vi "LVClass_HasoData Reset To RAW data.vi"(0 "HasoData in":refnum<class "HasoData.lvclass">, 11 "error in (no error)":errorcluster) -> (4 "HasoData out":refnum<class "HasoData.lvclass">, 15 "error out":errorcluster)   [LabVIEW 2020, in "HasoData.lvclass"]
doc: "Reset slopes to their raw state and clear process history.\n\n--------------------------------------------------------------------------------\n\n<B>HasoDataIn </B> : HasoData object.\n<B>HasoDataOut </B> : HasoData object.\n<B>ErrorIn </B> : Error\n<B>ErrorOut </B> : Error\n\n--------------------------------------------------------------------------------"
uses:
  HasoData.lvclass
  HasoData.lvclass/HasoData.ctl
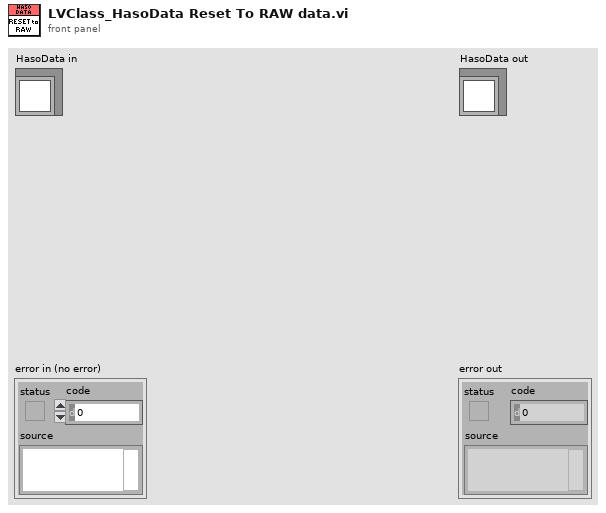
[diagram p1: front panel]
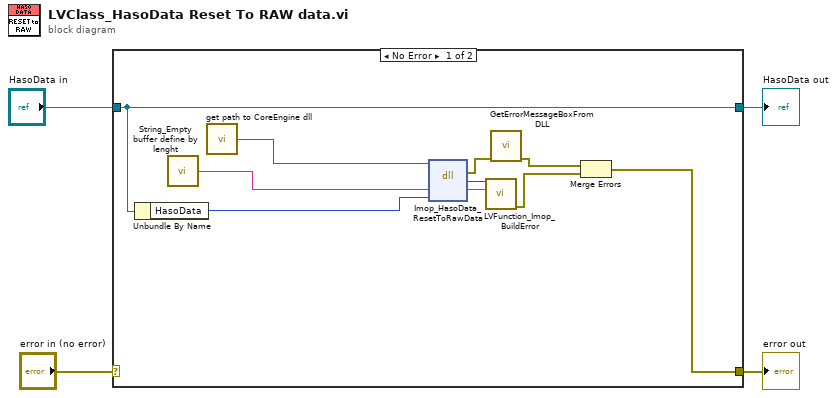
[diagram p0: block diagram]
diagram:
  n1 = case shown="No Error" "error in (no error)" {
    selector: "error in (no error)" -> [_ w16]
    tunnel: [w5 w16] -> w2
    tunnel: [w10 w15] -> w1
    tunnel: "HasoData in" -> [w10 w15]
    frame No Error {
      n2 = Unbundle By Name(w10) -> ("HasoData"=w11:i32)
      n3 = call "String_Empty buffer define by lenght.vi"() -> ("Empty buffer"=w12:string)  [unwired: 1 in]
      n4 = call "get path to CoreEngine dll.vi"() -> ("path to c_interface_vc100.dll"=w9:path)  [unwired: 12 in, 3 out]
      n5 = dll-call lib="D:/2_trunk/Soft_haso/ImOpCoreEngine4_LV2011/DLLs/ImopEngine4_vc100.dll" fn="Imop_HasoData_ResetToRawData"(path in=w9, "message"=w12, "objet"=w11) -> (error out=w8:errorcluster, "return type"=w14:i32, "message"=w13:string)  [unwired: 3 in, 1 out]
      n6 = call "LVFunction_Imop_BuildError.vi"("code"=w14, "String to Prepend to source (\"\")"=w13) -> ("error out"=w6:errorcluster)  [unwired: 13 in]
      n7 = call "GetErrorMessageBoxFromDLL.vi"("error IN"=w8) -> ("error OUT"=w7:errorcluster)  [unwired: 10 in]
      n8 = Merge Errors(w7, w6) -> (w5:errorcluster)
    }
    frame Error {
    }
  }
  "error out" <- w2
  "HasoData out" <- w1
